vi "Load Simple Explorer.vi"(8 "error in (no error)":errorcluster, 11 "Item Ref in":T2 format="%.0x") -> (0 "error out":errorcluster, 3 "Item Ref out":T2 format="%.0x")   [LabVIEW 2017, in "DSF System Explorer.lvlib"]
uses:
  DSF System Explorer.lvlib
  <vilib>/NI Veristand/Custom Device API/Custom Device Item Ref.ctl
  DSF Core.lvlibp/Classes/Configuration/Configuration Session.lvclass
  Development Tools/Data Sharing Configuration Explorer/Source/Item Tree/ID to Tree Items/Tree Item Type.ctl
  <vilib>/NI Veristand/Custom Device API/Get Item Property (String).vi
  <vilib>/NI Veristand/Custom Device API/Custom Device API.lvlib
  Development Tools/Data Sharing Configuration Explorer/DSF Configuration Utility.lvlib
panel:
  in  "Item Type":T1
  out "reference out":refnum<vi>
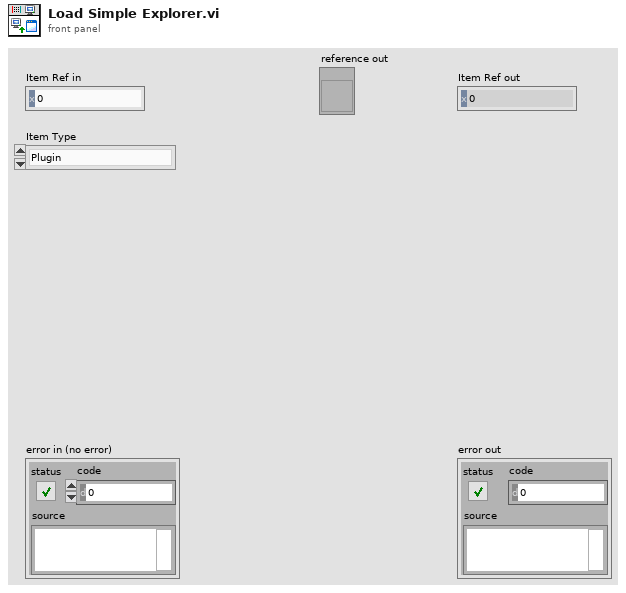
[diagram p1: front panel]
types:
  T1 = typedef "DSF Configuration Utility.lvlib/Tree Item Type.ctl" = enum16{"Plugin", "Group", "Transfer", "Channel", "Setting"}
  T2 = typedef "Custom Device API.lvlib/Custom Device Item Ref.ctl" = u64
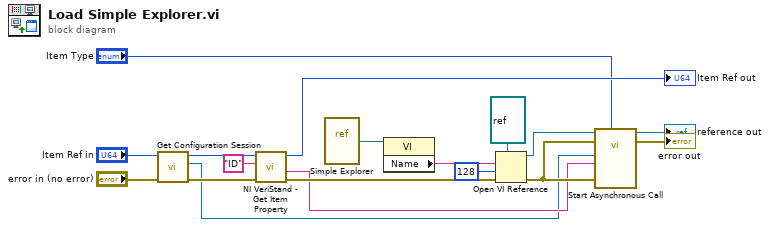
[diagram p0: block diagram]
diagram:
  n1 = call "Get Configuration Session.vi"("error in (no error)"="error in (no error)", "Item Ref in"="Item Ref in") -> ("error out"=w7:errorcluster, "Configuration Session"=w3:refnum<class "Configuration Session.lvclass">, "Item Ref out"=w8:T2)  [unwired: 7 in]
  n2 = call-poly <vilib>:"NI VeriStand - Get Item Property.vi"("error in (no error)"=w7, "Property Name"="ID", "Item Ref in"=w8) -> ("error out"=w6:errorcluster, "Value"=w4:string, "Item Ref out"=→"Item Ref out":T2)  [unwired: 5 in, 1 out]
  n3 = vi-ref "Simple Explorer.vi"() -> (w15:refnum<vi>)
  n4 = property class="VI"(reference=w15) -> ("Name"=w14:string)  [unwired: 1 in, 2 out]
  n5 = Open VI Reference(type specifier VI Refnum (for type only)=refnum<vi> refnum, vi path=w14, options=128, error in (no error)=w6) -> (vi reference=w12:refnum<vi>, error out=w16:errorcluster)  [unwired: 2 in]
  n6 = call-by-ref "Start Asynchronous Call"(reference=w12, error in=w16, "Item Type"="Item Type", 8:"error in (no error)"=w16, "Item ID"=w4, "Configuration Session"=w3) -> (reference out=→"reference out":refnum<vi>, error out=→"error out":errorcluster)  [unwired: 7 in, 1 out]
